vi "Explorer - Populate (SubVI).vi"(6 "Asc?":bool=TRUE, 7 "TreeDone":refnum<vi>, 8 "error in (no error)":errorcluster, 9 "Test Data":string, 10 "TreeRun":refnum<vi>, 11 "RefIn":T1) -> (0 "error out":errorcluster, 1 "TestName Done":string[](array[string]), 2 "TestName Running":string[](array[string]), 3 "Refnum out":T1, 4 "Name Done":string[](array[string]), 5 "Name Running":string[](array[string]))   [LabVIEW 2019]
uses:
  <vilib>/httpClient/ClientHandle.ctl
  Controls/JSON - Fileid.ctl
  Controls/JSON - Stage.ctl
  <vilib>/httpClient/POSTBuffer.vi
  <vilib>/httpClient/LabVIEWHTTPClient.lvlib
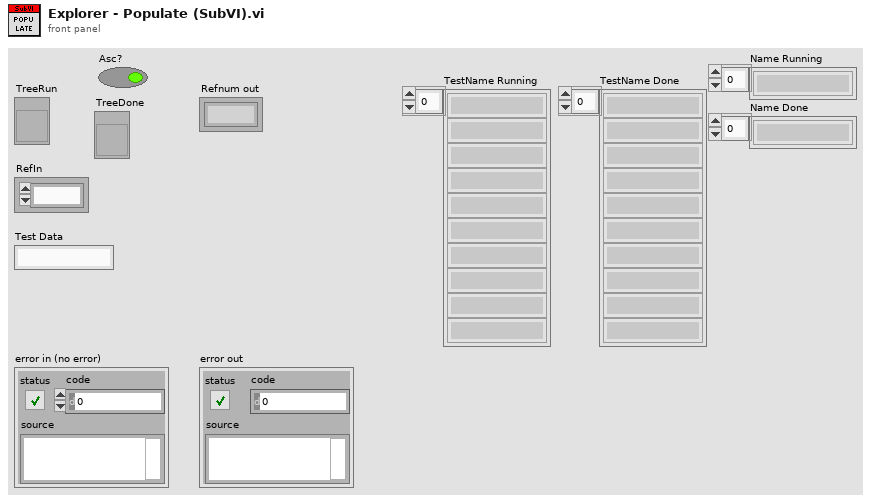
[diagram p1: front panel]
types:
  T1 = typedef "LabVIEWHTTPClient.lvlib/ClientHandle.ctl" = refnum<k1>
  T2 = typedef "JSON - Fileid.ctl" = cluster{"status":string, "data":cluster{"id":string, "created_date":string, "testname":string, "jobno":string, "jobdesc":string, "sampleid":string, "date":string, "specimentno":string, "depth":string, "height":string, "diameter":string, "weight":string, "done":string}[]}
  T3 = cluster{"id":string, "created_date":string, "testname":string, "jobno":string, "jobdesc":string, "sampleid":string, "date":string, "specimentno":string, "depth":string, "height":string, "diameter":string, "weight":string, "done":string}[]
  T4 = typedef "JSON - Stage.ctl" = cluster{"status":string, "data":cluster{"id":string, "created_date":string, "filename":string, "stage":string, "testplan":string, "station":string, "status":string, "delete":string}[]}
  T5 = cluster{"id":string, "created_date":string, "filename":string, "stage":string, "testplan":string, "station":string, "status":string, "delete":string}[]
  T6 = cluster{"TestPlan Section":string, "Key Value":string[]}[]
  T7 = cluster{"TestPlan Section":string, "Key Value":string[]}
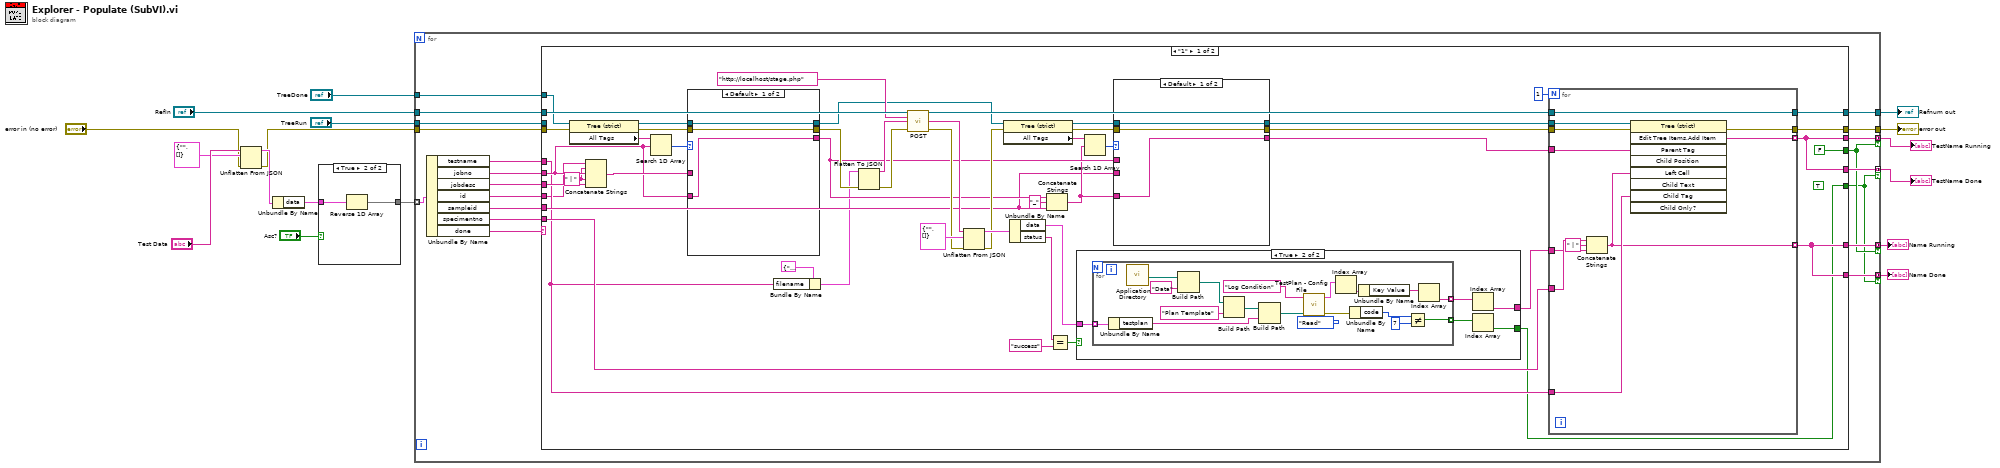
[diagram p0: block diagram]
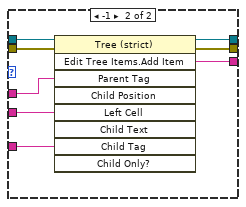
[diagram p3: hidden frame]
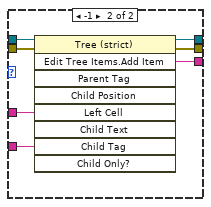
[diagram p4: hidden frame]
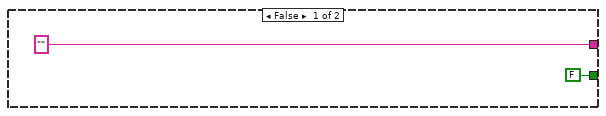
[diagram p5: hidden frame]
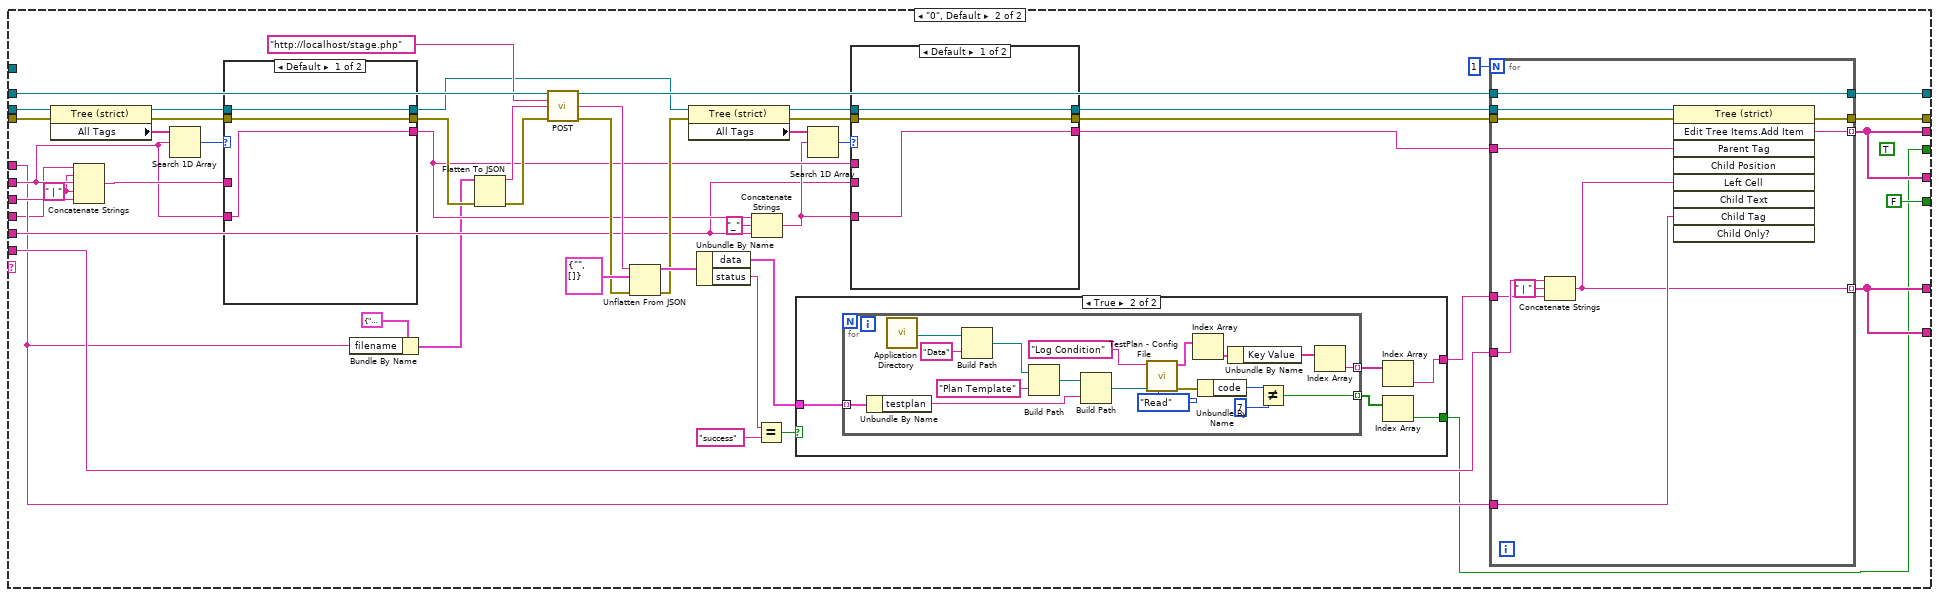
[diagram p6: hidden frame]
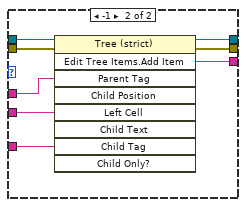
[diagram p7: hidden frame]
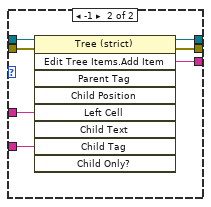
[diagram p8: hidden frame]
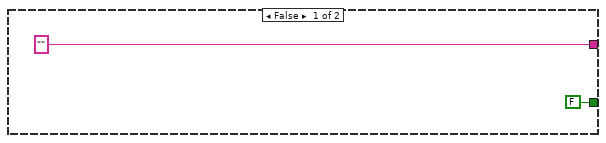
[diagram p9: hidden frame]
diagram:
  n1 = Unflatten From JSON(JSON string="Test Data", type and defaults=T2 {"status"="", "data"=[]}, error in (no error)="error in (no error)") -> (value=w12:T2, error out=w9:errorcluster)  [unwired: 4 in]
  n2 = Unbundle By Name(w12) -> ("data"=w14:T3)
  n3 = case shown="True" "Asc?" {
    tunnel: w14 -> [w18 w20]
    tunnel: [w18 w19] -> w8
    frame False {
    }
    frame True {
      n4 = Reverse 1D Array(array=w20) -> (reversed array=w19:T3)
    }
  }
  n5 = for {
    tunnel: w9 -> [w36]
    tunnel: "RefIn" -> [w37]
    tunnel: w8 -> [w40] mode=indexing
    tunnel: [w38] -> w17
    tunnel: [w39] -> w15
    tunnel: "TreeRun" -> [w31]
    tunnel: "TreeDone" -> [w28]
    tunnel: [w27] -> w5 mode=concatenating if=w23
    tunnel: [w26] -> w4 mode=concatenating if=w22
    tunnel: [w25] -> w3 mode=concatenating if=w23
    tunnel: [w24] -> w2 mode=concatenating if=w22
    n6 = Unbundle By Name(w40) -> ("testname"=w21:string, "jobno"=w35:string, "jobdesc"=w34:string, "id"=w30:string, "sampleid"=w33:string, "specimentno"=w32:string, "done"=w29:string)
    n7 = case shown="\"1\"" w29 {
      tunnel: [w79 w186] -> w39
      tunnel: [w76 w183] -> w38
      tunnel: w37 -> [w74 w181]
      tunnel: w36 -> [w67 w174]
      tunnel: w35 -> [w63 w171]
      tunnel: w34 -> [w73 w180]
      tunnel: w33 -> [w51 w159]
      tunnel: w32 -> [w72 w179]
      tunnel: w31 -> [_ w153]
      tunnel: w30 -> [w41 w148]
      tunnel: [w43 FALSE] -> w22
      tunnel: [FALSE w150] -> w23
      tunnel: w28 -> [w65 _]
      tunnel: w21 -> [w48 w156]
      tunnel: [w50 w158] -> w27
      tunnel: [w50 w158] -> w26
      tunnel: [w45 w152] -> w25
      tunnel: [w45 w152] -> w24
      frame "1" {
        (unwired) TRUE
        w42 = " | " ("string")
        n8 = property class="Tree (strict)"(reference=w65, error in=w67) -> (reference out=w66:refnum<vi>, error out=w68:errorcluster, "All Tags"=w64:string[])
        n9 = Concatenate Strings(w41, w42, w63, w42, w73) -> (w75:string)
        n10 = Search 1D Array(1D array=w64, element=w63) -> (index of element=w62:i32)  [unwired: 1 in]
        n11 = case shown="Default" w62 {
          tunnel: [w103 w111] -> w89
          tunnel: [w102 w105] -> w54
          tunnel: w75 -> [_ w110]
          tunnel: [w104 w109] -> w60
          tunnel: w66 -> [w104 w108]
          tunnel: w63 -> [w102 w107]
          tunnel: w68 -> [w103 w106]
          frame Default {
          }
          frame -1 {
            n12 = invoke on="Invoke Node" class="Tree (strict)" method="Edit Tree Items.Add Item"(reference=w108, error in=w106, "Left Cell"=w110, "Child Tag"=w107) -> (reference out=w109:refnum<vi>, error out=w111:errorcluster, "Edit Tree Items:Add Item"=w105:string)  [unwired: 5 in, 6 out]
          }
        }
        n13 = Bundle By Name(cluster=cluster{"filename":string, "action":string} {"filename"="", "action"="read"}, "filename"=w48) -> (w47:cluster{"filename":string, "action":string})
        n14 = Flatten To JSON(anything=w47, error in (no error)=w89) -> (JSON string=w87:string, 11:w88:errorcluster)  [unwired: 1 in]
        n15 = call-poly <vilib>:"POST.vi"("client handle"=w74, "url"="http://localhost/stage.php", "buffer"=w87, "error in (no error)"=w88) -> ("client handle out"=w78:T1, "body"=w81:string, "error out"=w80:errorcluster)  [unwired: 8 in, 1 out]
        n16 = Unflatten From JSON(JSON string=w81, type and defaults=T4 {"status"="", "data"=[]}, error in (no error)=w80) -> (value=w84:T4, error out=w58:errorcluster)  [unwired: 4 in]
        n17 = property class="Tree (strict)"(reference=w60, error in=w58) -> (reference out=w59:refnum<vi>, error out=w57:errorcluster, "All Tags"=w61:string[])
        n18 = Unbundle By Name(w84) -> ("data"=w55:T5, "status"=w85:string)
        n19 = Concatenate Strings(w54, "_" ("string"), w51) -> (w52:string)
        n20 = Equal?(x=w85, y="success") -> (x = y?=w86:bool)
        n21 = case shown="True" w86 {
          tunnel: w55 -> [_ w129]
          tunnel: ["" w127] -> w46
          tunnel: [FALSE w125] -> w43
          frame False {
          }
          frame True {
            n22 = for {
              tunnel: w129 -> [w147] mode=indexing
              tunnel: [w134] -> w128 mode=indexing
              tunnel: [w130] -> w126 mode=indexing
              n23 = Unbundle By Name(w147) -> ("testplan"=w136:string)
              n24 = call <vilib>:"Application Directory.vi"() -> ("Application Directory"=w142:path)
              n25 = Build Path(base path=w142, name or relative path="Data") -> (appended path=w143:path)
              n26 = Build Path(base path=w143, name or relative path="Plan Template") -> (appended path=w141:path)
              n27 = Build Path(base path=w141, name or relative path=w136) -> (appended path=w146:path)
              n28 = call "TestPlan - Config File.vi"("Action"=enum16{"Write", "Read", "Read All", "Remove"}."Read", "file path"=w146, "TestPlan Section"="Log Condition") -> ("error out"=w133:errorcluster, "Value Out"=w144:T6)  [unwired: 6 in, 1 out]
              n29 = Index Array(array=w144) -> (element=w145:T7)  [unwired: 1 in]
              n30 = Unbundle By Name(w133) -> ("code"=w132:i32)
              n31 = Unbundle By Name(w145) -> ("Key Value"=w135:string[])
              n32 = Not Equal?(x=w132, y=7) -> (x != y?=w130:bool)
              n33 = Index Array(array=w135) -> (element=w134:string)  [unwired: 1 in]
            }
            n34 = Index Array(array=w128) -> (element=w127:string)  [unwired: 1 in]
            n35 = Index Array(array=w126) -> (element=w125:bool)  [unwired: 1 in]
          }
        }
        n36 = Search 1D Array(1D array=w61, element=w52) -> (index of element=w56:i32)  [unwired: 1 in]
        n37 = case shown="Default" w56 {
          tunnel: [w92 w101] -> w90
          tunnel: [w91 w100] -> w77
          tunnel: w54 -> [_ w95]
          tunnel: [w93 w99] -> w71
          tunnel: w52 -> [w91 w98]
          tunnel: w59 -> [w93 w97]
          tunnel: w57 -> [w92 w96]
          tunnel: w51 -> [_ w94]
          frame Default {
          }
          frame -1 {
            n38 = invoke on="Invoke Node" class="Tree (strict)" method="Edit Tree Items.Add Item"(reference=w97, error in=w96, "Parent Tag"=w95, "Left Cell"=w94, "Child Tag"=w98) -> (reference out=w99:refnum<vi>, error out=w101:errorcluster, "Edit Tree Items:Add Item"=w100:string)  [unwired: 4 in, 6 out]
          }
        }
        n39 = for {
          N: 1 -> [_]
          tunnel: w90 -> [w122]
          tunnel: w77 -> [w121]
          tunnel: w46 -> [w114]
          tunnel: [w119] -> w76
          tunnel: [w118] -> w79
          tunnel: w78 -> [w118]
          tunnel: w72 -> [w117]
          tunnel: w71 -> [w116]
          tunnel: w48 -> [w115]
          tunnel: [w113] -> w50 mode=indexing
          tunnel: [w112] -> w45 mode=indexing
          n40 = Concatenate Strings(w117, " | " ("string"), w114) -> (w112:string)
          n41 = invoke on="Invoke Node" class="Tree (strict)" method="Edit Tree Items.Add Item"(reference=w116, error in=w122, "Parent Tag"=w121, "Left Cell"=w112, "Child Tag"=w115) -> (error out=w119:errorcluster, "Edit Tree Items:Add Item"=w113:string)  [unwired: 4 in, 7 out]
        }
      }
      frame "0", Default {
        (unwired) TRUE
        w149 = " | " ("string")
        n42 = property class="Tree (strict)"(reference=w153, error in=w174) -> (reference out=w173:refnum<vi>, error out=w175:errorcluster, "All Tags"=w172:string[])
        n43 = Concatenate Strings(w148, w149, w171, w149, w180) -> (w182:string)
        n44 = Search 1D Array(1D array=w172, element=w171) -> (index of element=w170:i32)  [unwired: 1 in]
        n45 = case shown="Default" w170 {
          tunnel: [w210 w218] -> w196
          tunnel: [w209 w212] -> w162
          tunnel: w182 -> [_ w217]
          tunnel: [w211 w216] -> w168
          tunnel: w173 -> [w211 w215]
          tunnel: w171 -> [w209 w214]
          tunnel: w175 -> [w210 w213]
          frame Default {
          }
          frame -1 {
            n46 = invoke on="Invoke Node" class="Tree (strict)" method="Edit Tree Items.Add Item"(reference=w215, error in=w213, "Left Cell"=w217, "Child Tag"=w214) -> (reference out=w216:refnum<vi>, error out=w218:errorcluster, "Edit Tree Items:Add Item"=w212:string)  [unwired: 5 in, 6 out]
          }
        }
        n47 = Bundle By Name(cluster=cluster{"filename":string, "action":string} {"filename"="", "action"="read"}, "filename"=w156) -> (w155:cluster{"filename":string, "action":string})
        n48 = Flatten To JSON(anything=w155, error in (no error)=w196) -> (JSON string=w194:string, 11:w195:errorcluster)  [unwired: 1 in]
        n49 = call-poly <vilib>:"POST.vi"("client handle"=w181, "url"="http://localhost/stage.php", "buffer"=w194, "error in (no error)"=w195) -> ("client handle out"=w185:T1, "body"=w188:string, "error out"=w187:errorcluster)  [unwired: 8 in, 1 out]
        n50 = Unflatten From JSON(JSON string=w188, type and defaults=T4 {"status"="", "data"=[]}, error in (no error)=w187) -> (value=w191:T4, error out=w166:errorcluster)  [unwired: 4 in]
        n51 = property class="Tree (strict)"(reference=w168, error in=w166) -> (reference out=w167:refnum<vi>, error out=w165:errorcluster, "All Tags"=w169:string[])
        n52 = Unbundle By Name(w191) -> ("data"=w163:T5, "status"=w192:string)
        n53 = Concatenate Strings(w162, "_" ("string"), w159) -> (w160:string)
        n54 = Equal?(x=w192, y="success") -> (x = y?=w193:bool)
        n55 = case shown="True" w193 {
          tunnel: w163 -> [_ w236]
          tunnel: ["" w234] -> w154
          tunnel: [FALSE w232] -> w150
          frame False {
          }
          frame True {
            n56 = for {
              tunnel: w236 -> [w254] mode=indexing
              tunnel: [w241] -> w235 mode=indexing
              tunnel: [w237] -> w233 mode=indexing
              n57 = Unbundle By Name(w254) -> ("testplan"=w243:string)
              n58 = call <vilib>:"Application Directory.vi"() -> ("Application Directory"=w249:path)
              n59 = Build Path(base path=w249, name or relative path="Data") -> (appended path=w250:path)
              n60 = Build Path(base path=w250, name or relative path="Plan Template") -> (appended path=w248:path)
              n61 = Build Path(base path=w248, name or relative path=w243) -> (appended path=w253:path)
              n62 = call "TestPlan - Config File.vi"("Action"=enum16{"Write", "Read", "Read All", "Remove"}."Read", "file path"=w253, "TestPlan Section"="Log Condition") -> ("error out"=w240:errorcluster, "Value Out"=w251:T6)  [unwired: 6 in, 1 out]
              n63 = Index Array(array=w251) -> (element=w252:T7)  [unwired: 1 in]
              n64 = Unbundle By Name(w240) -> ("code"=w239:i32)
              n65 = Unbundle By Name(w252) -> ("Key Value"=w242:string[])
              n66 = Not Equal?(x=w239, y=7) -> (x != y?=w237:bool)
              n67 = Index Array(array=w242) -> (element=w241:string)  [unwired: 1 in]
            }
            n68 = Index Array(array=w235) -> (element=w234:string)  [unwired: 1 in]
            n69 = Index Array(array=w233) -> (element=w232:bool)  [unwired: 1 in]
          }
        }
        n70 = Search 1D Array(1D array=w169, element=w160) -> (index of element=w164:i32)  [unwired: 1 in]
        n71 = case shown="Default" w164 {
          tunnel: [w199 w208] -> w197
          tunnel: [w198 w207] -> w184
          tunnel: w162 -> [_ w202]
          tunnel: [w200 w206] -> w178
          tunnel: w160 -> [w198 w205]
          tunnel: w167 -> [w200 w204]
          tunnel: w165 -> [w199 w203]
          tunnel: w159 -> [_ w201]
          frame Default {
          }
          frame -1 {
            n72 = invoke on="Invoke Node" class="Tree (strict)" method="Edit Tree Items.Add Item"(reference=w204, error in=w203, "Parent Tag"=w202, "Left Cell"=w201, "Child Tag"=w205) -> (reference out=w206:refnum<vi>, error out=w208:errorcluster, "Edit Tree Items:Add Item"=w207:string)  [unwired: 4 in, 6 out]
          }
        }
        n73 = for {
          N: 1 -> [_]
          tunnel: w197 -> [w229]
          tunnel: w184 -> [w228]
          tunnel: w154 -> [w221]
          tunnel: [w226] -> w183
          tunnel: [w225] -> w186
          tunnel: w185 -> [w225]
          tunnel: w179 -> [w224]
          tunnel: w178 -> [w223]
          tunnel: w156 -> [w222]
          tunnel: [w220] -> w158 mode=indexing
          tunnel: [w219] -> w152 mode=indexing
          n74 = Concatenate Strings(w224, " | " ("string"), w221) -> (w219:string)
          n75 = invoke on="Invoke Node" class="Tree (strict)" method="Edit Tree Items.Add Item"(reference=w223, error in=w229, "Parent Tag"=w228, "Left Cell"=w219, "Child Tag"=w222) -> (error out=w226:errorcluster, "Edit Tree Items:Add Item"=w220:string)  [unwired: 4 in, 7 out]
        }
      }
    }
  }
  "error out" <- w17
  "Refnum out" <- w15
  "TestName Done" <- w4
  "TestName Running" <- w5
  "Name Running" <- w3
  "Name Done" <- w2
